vi "Testing Mode.vi"(8 "Filepath":path=path "D:/My Project/2019-2020/Magnetic Mareli UM/MM_UM/Project Setup/data/program seq/Program_280A.bin", 9 "FeedBack Channel":string[](array[string])=["fgdgfvcbc", "vnfhgjkn", "21354682"]) -> ()   [LabVIEW 2015]
uses:
  Control Button/Exit.ctl
  Control Button/Start.ctl
  Test  enqueue/AutoTest seq.ctl
  Test  enqueue/Auot Test selection.ctl
  Galobal variable_TI.vi
  Project Setup/Globle Variable/GR_Servo.vi
  <vilib>/Utility/file.llb/Write Delimited Spreadsheet (string).vi
panel:
  out "Ready":bool
  in  "Seq1":enum16{"Seq_1", "Seq_2", "Seq_3", "Seq_4"}(ring)
  out "Dist. data":dbl[](array[numeric]) format="%0.03f"
  out "Proxi Sensor":bool
  in  "value":bool
  out "reset":bool
  out "D-enqueue":T1
  out "Servo Fault":bool
  in  "Report":bool
  out "Start":bool
  in  "Cycle":i32
  in  "Home Call":bool
  out "DI":bool[](array[boolean])
  out "Current Date & Time":timestamp
  in  "Cycle Start Bit":bool
  in  "vi reference":refnum<vi>
  in  "Reset Ct.":bool
  out "error out":errorcluster
  in  "Tbl Refnum":refnum<vi>
  in  "Tab Control":enum32{"Test", "Report"}(tab)
  out "RR":bool
  out "RL":bool
  out "FR":bool
  out "FL":bool
  out "Error Message 2":string
  out "User Name":string
  out "Error Message":string
  out "Running Model":string
  out "Date time":string
  out "MIC Barcode":string
  out "2D Picture":picture
  out "Screw Data(N)":T2
  in  "Tab Control 2":enum32{"TESTING", "HOME"}(tab)
  in  "Table Control":string[][](table)
  in  "home":string[][](table)
  out "Error":bool
  out "Read LVDT Value":dbl[](array[numeric]) format="%0.03f"
  out "Result Lvdt 2":T3 {"Screw4(mm)" format="%0.02f"; "Screw3(mm)" format="%0.02f"; "Screw 2(mm)" format="%0.02f"; "Screw1(mm)" format="%0.02f"}
  out "Result Lvdt":T4
  out "Test Name":string
  in  "Exit":T5
  in  "Start 2":T6
  out "Cycle Time(Sec)":i32
  out "MIC Code":string
  in  "OK Counter":string
  in  "NG Counter":string
  in  "RPT Bypass":bool=TRUE
  out "Pokayoka":T7
  out "Boolean 2":bool
  in  "Report":i32(listbox)
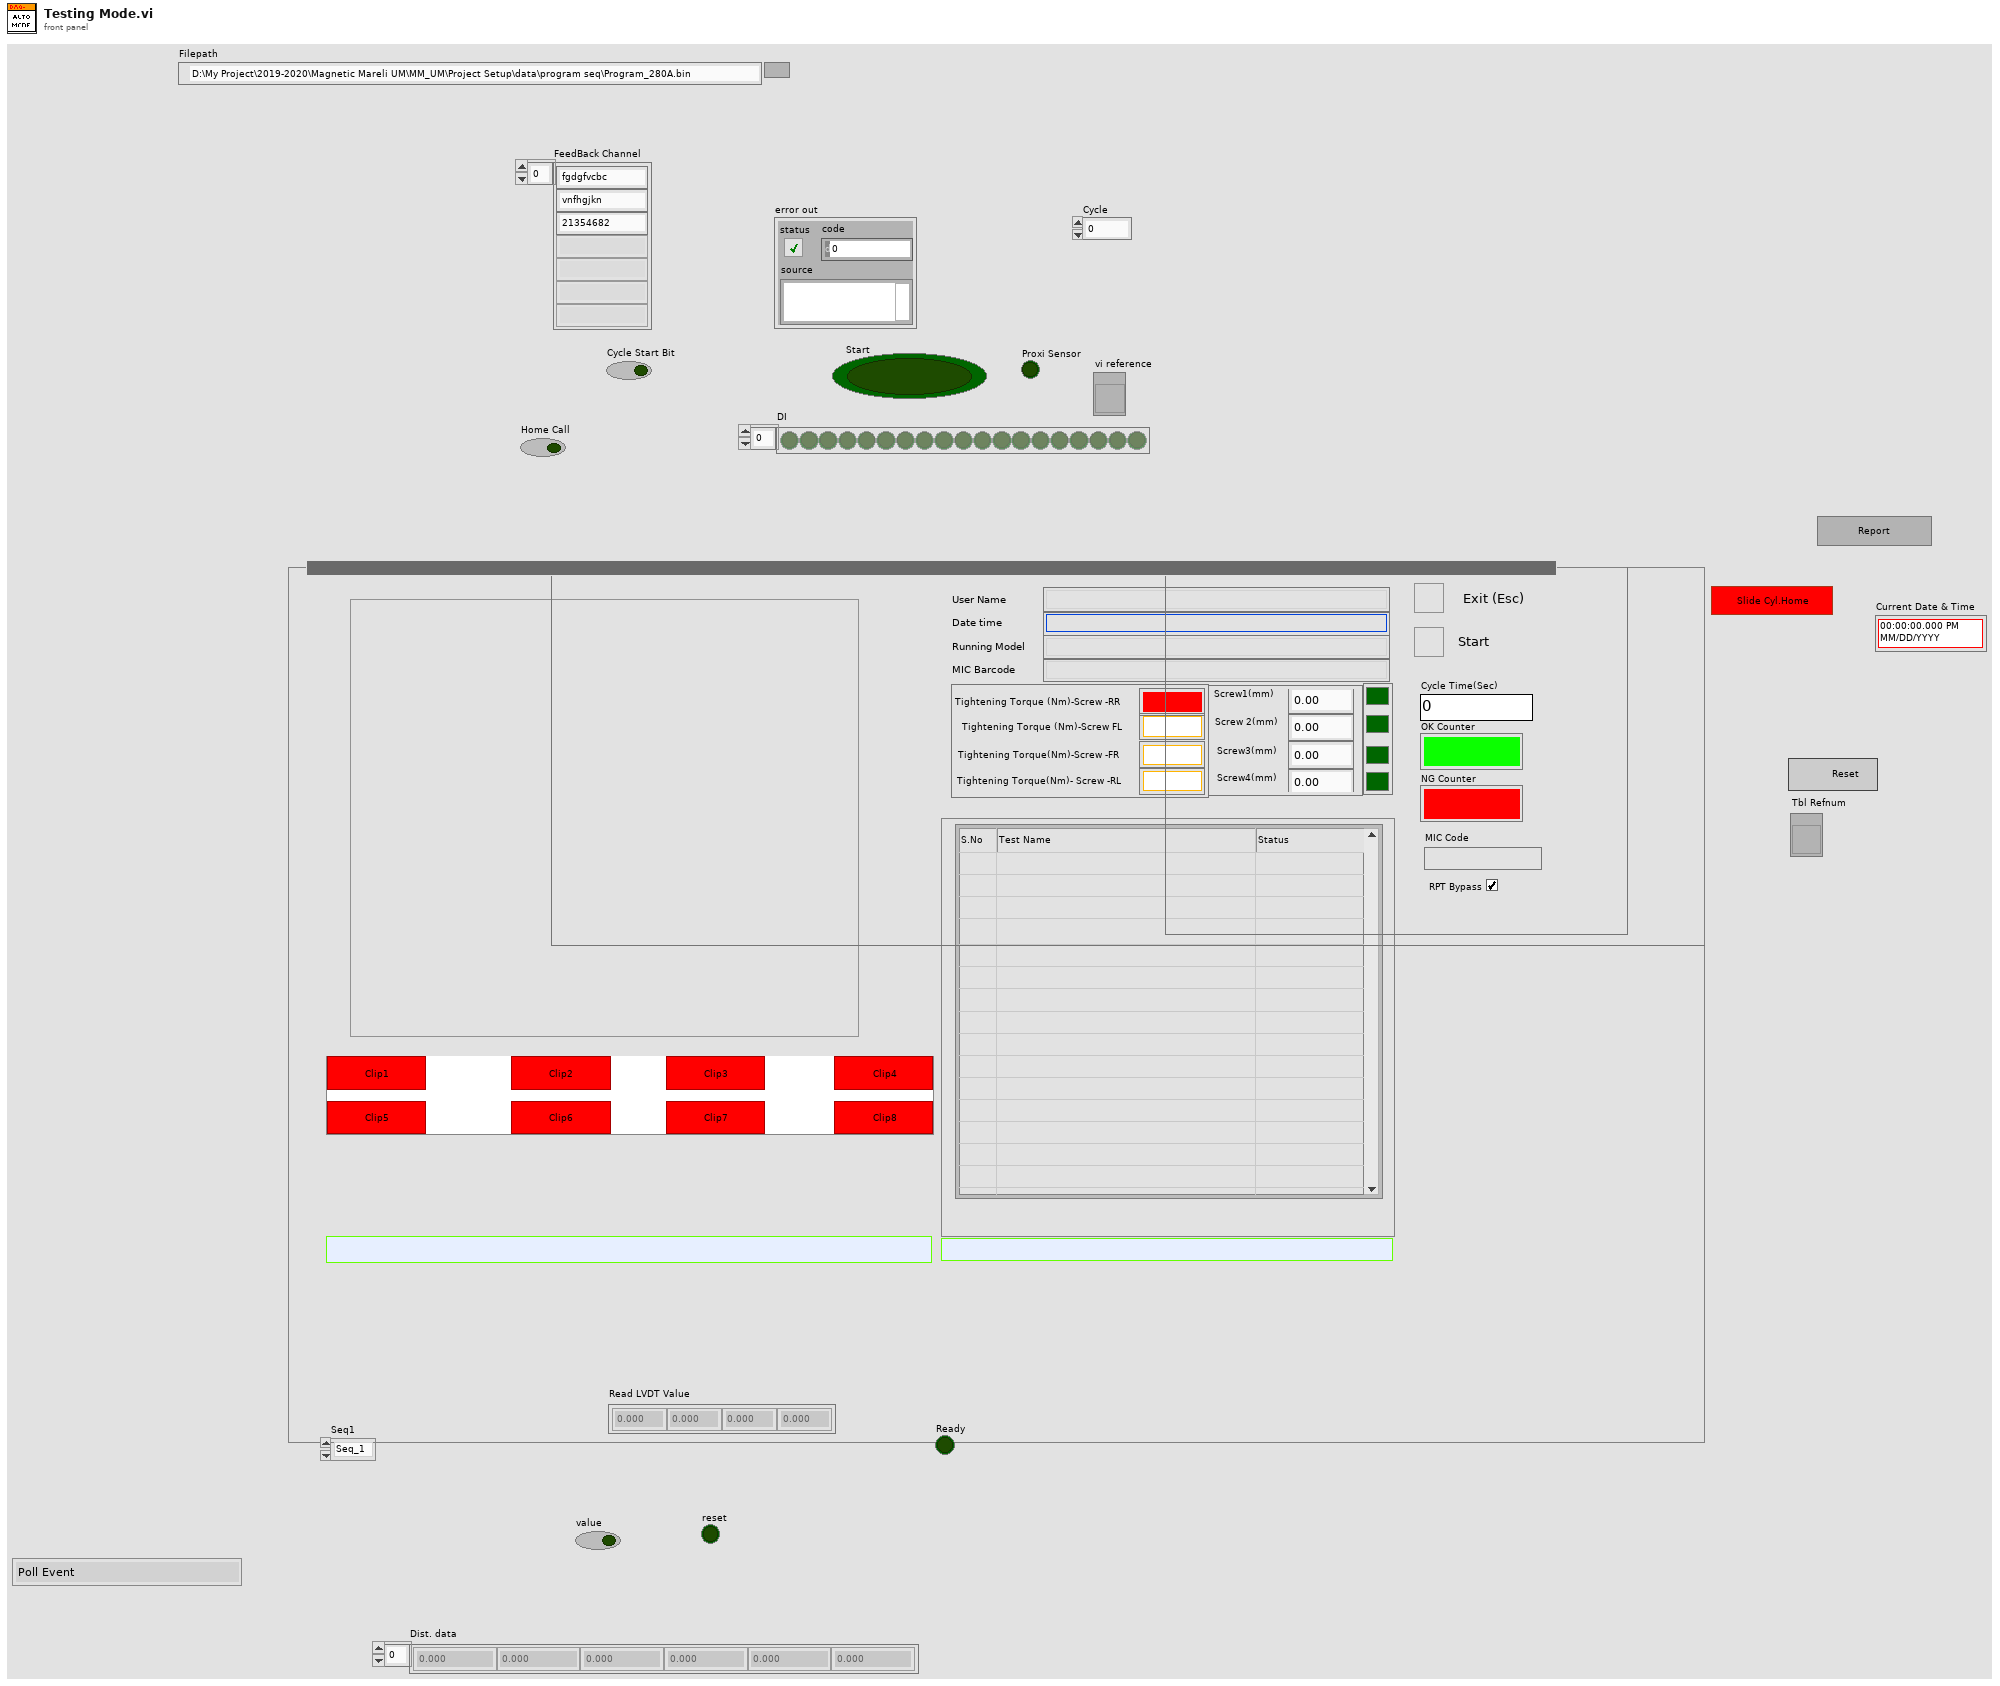
[diagram p1: front panel]
types:
  T1 = typedef "AutoTest seq.ctl" = enum16{"Poll Event", "Part Clamp", "Program Seq", "Cylender Home", "Result Save", "Error", "Exit"}
  T2 = cluster{"Tightening Torque (Nm)-Screw -RR":string, "Tightening Torque (Nm)-Screw FL ":string, "Tightening Torque(Nm)-Screw -FR":string, "Tightening Torque(Nm)- Screw -RL":string}
  T3 = cluster{"Screw1(mm)":dbl, "Screw 2(mm)":dbl, "Screw3(mm)":dbl, "Screw4(mm)":dbl}
  T4 = cluster{"Screw Height-1":bool, "Screw Height-2":bool, "Screw Height-3":bool, "Screw Height-4":bool}
  T5 = typedef "Exit.ctl" = bool
  T6 = typedef "Start.ctl" = bool
  T7 = cluster{"Clip1":bool, "Clip2 3":bool, "Clip3 3":bool, "Clip4":bool, "Clip5":bool, "Clip6":bool, "Clip7":bool, "Clip8":bool}
  T8 = cluster{"Screw -FL":string, "Screw -FR":string, "Screw -RL":string, "Screw -RR":string}
  T9 = cluster{"MIC ":refnum<visa-resource-name>, "baud rate MIC ":u32, "LCD ":refnum<visa-resource-name>, "baud rate_LCD":u32}
  T10 = typedef "Auot Test selection.ctl" = enum16{"Init", "Enqueue ", "Enqueue N", "Enqueue in stack", "Enqueue in stack N", "Dequeue", "Dequeue N", "Flush", "Release Queue"}
  T11 = cluster{"LVDT1Max(mm) AI0":dbl, "LVDT1Min (mm)AI0":dbl, "LVDT2Max(mm) AI1":dbl, "LVDT2Min(mm) AI1":dbl, "LVDT3Max(mm) AI2":dbl, "LVDT3Min(mm) AI2":dbl, "LVDT4Max(mm) AI3":dbl, "LVDT4Min(mm) AI3":dbl, "Model":string, "MIC Code":string}
  T12 = cluster{"Item Name":string, "Item Status":bool, "Steps":cluster{"Channel Type":string, "Channels":string, "Wait/Poll (ms)":u32, "Parameter":u8, "STM-Speed":i32, "STM-Degree":u32, "Direction":u8}[]}[]
  T13 = cluster{"Nuth Height1":bool, "Nuth Height2":bool, "Nuth Height3":bool, "Nuth Height4":bool}
  T14 = enum16{"Part Clamp", "Part Unclamp", "Part Clamp Input Check", "Part Unclamp Input Check"}
  T15 = cluster{"No. Fail Coun t":string, "Rework Status Count 0\\1":string, "NA Count Max =3 ":string, "Testesd Count  0/1":string, "Error code":string}
  T16 = cluster{"Emergency_1":bool, "Reset_2":bool, "Air Pressure_4":bool, "Safety Sensor_5":bool, "Safety Sensor_6":bool, "Barcode Rev rs_24":bool, "Clamp fwd rs_21":bool, "Servo Fault":bool, "Home _3":bool}
  T17 = cluster{"Read LVDT Value[0]":dbl, "Read LVDT Value[1]":dbl, "Read LVDT Value[2]":dbl, "Read LVDT Value[3]":dbl}
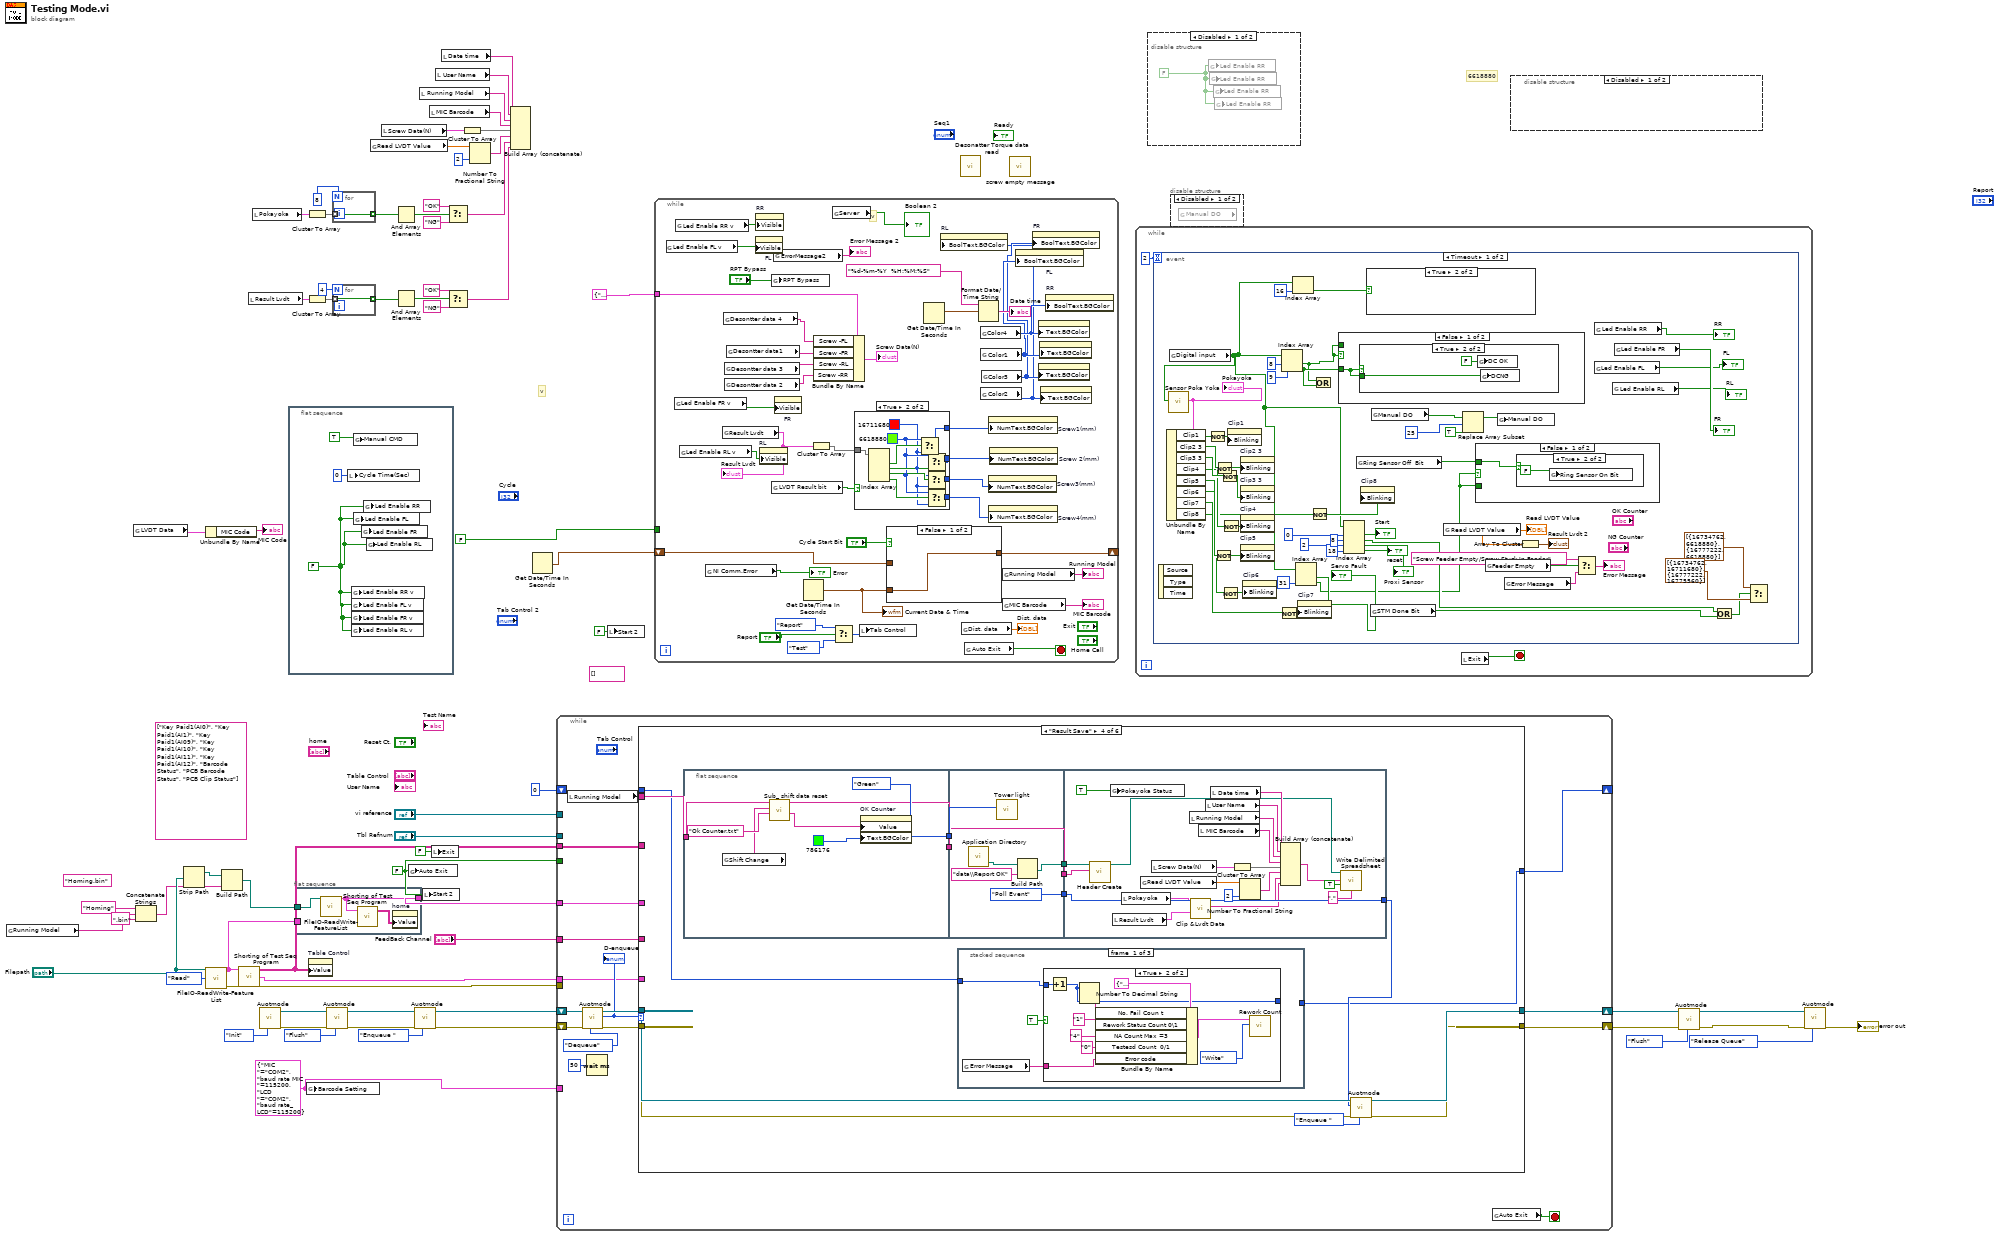
[diagram p0: block diagram]
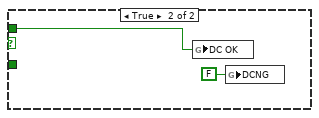
[diagram p7: hidden frame]
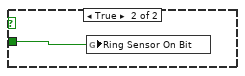
[diagram p9: hidden frame]
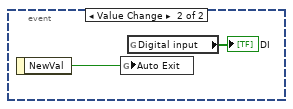
[diagram p10: hidden frame]
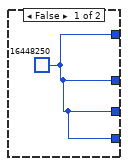
[diagram p11: hidden frame]
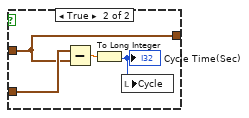
[diagram p12: hidden frame]
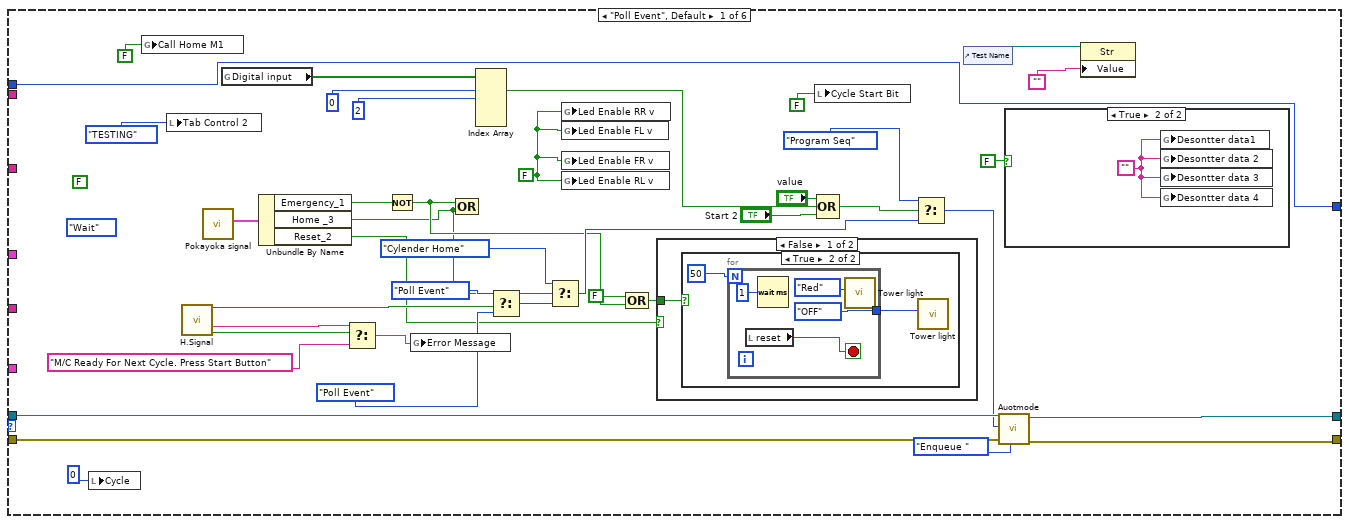
[diagram p13: hidden frame]
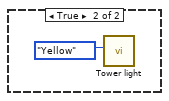
[diagram p16: hidden frame]
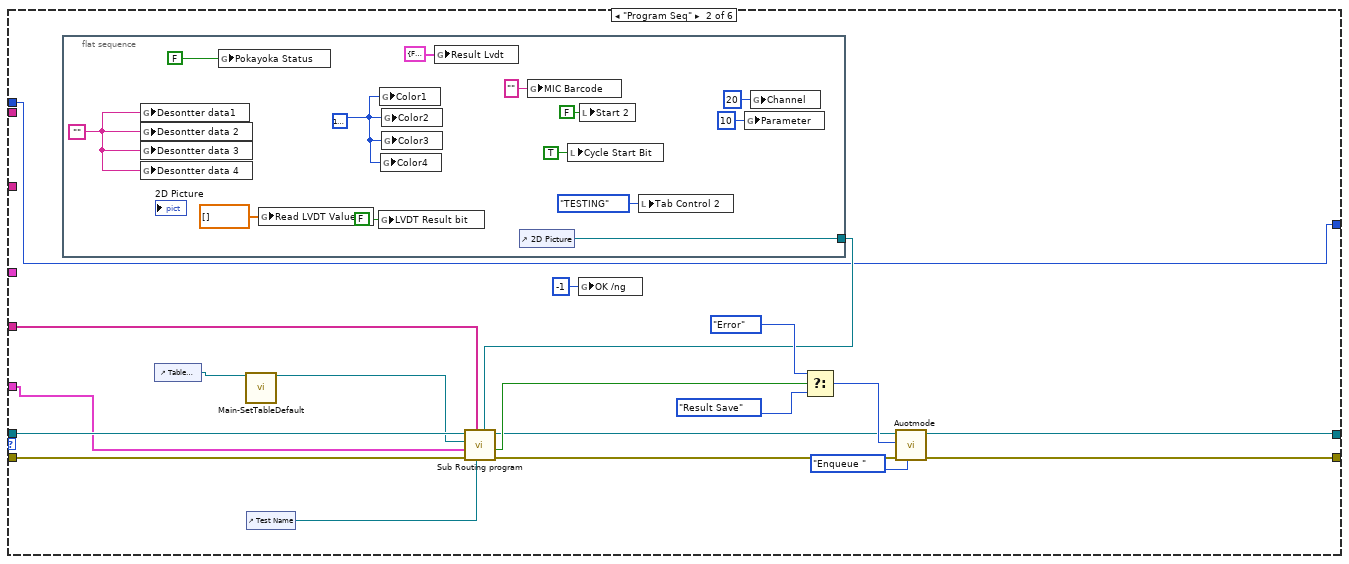
[diagram p17: hidden frame]
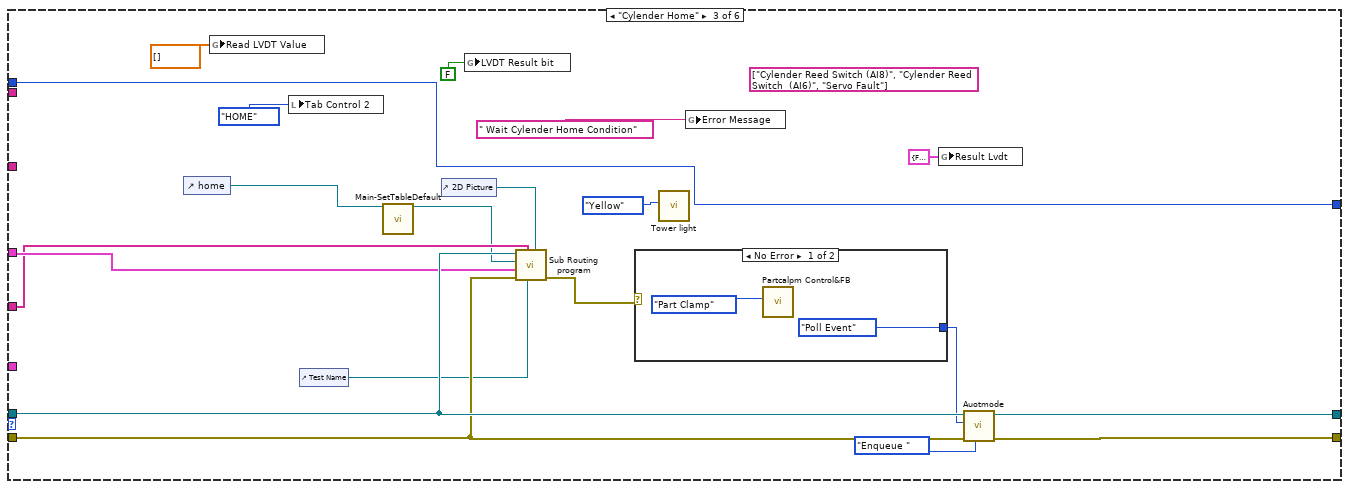
[diagram p18: hidden frame]
diagram:
  w34 = T9 {"MIC "="COM2", "baud rate MIC "=115200, "LCD "="COM2", "baud rate_LCD"=115200} ("Barcode Setting")
  (unwired) "Homing.bin" ("name or relative path")
  (unwired) string[] ["Key Paid1(AI0)", "Key Paid1(AI1)", "Key Paid1(AI09)", "Key Paid1(AI10)", "Key Paid1(AI11)", "Key Paid1(AI12)", "Barcode Status", "PCB Barcode Status", "PCB Clip Status"] ("Error Name")
  (unwired) string[] []
  w41 = FALSE ("Auto Exit")
  # "v"
  # "6618880"
  n1 = global read "Galobal variable_TI.vi" "Running Model"() -> (w32:string)
  n2 = global read "Galobal variable_TI.vi" "LVDT Data"() -> (w28:T11)
  n3 = Concatenate Strings("Homing" ("string"), w32, ".bin" ("string")) -> (w30:string)
  n4 = Strip Path(path="Filepath") -> (stripped path=w38:path)  [unwired: 1 out]
  n5 = Unbundle By Name(w28) -> ("MIC Code"=→"MIC Code":string)
  n6 = call "FileIO-ReadWrite-FeatureList.vi"("Filepath"="Filepath", "Read/Write"=enum16{"Read", "Write"}."Read") -> ("Feature List (Out)"=w36:T12, "Error Out"=w49:errorcluster)  [unwired: 12 in]
  n7 = Build Path(base path=w38, name or relative path=w30) -> (appended path=w37:path)
  n8 = call "Shorting of Test Seq Program.vi"("Feature List (Out)"=w36) -> ("Feature Step Enable"=w43:T12, "Feature Name"=w42:string[][])  [unwired: 3 in]
  n9 = local read "Result Lvdt"() -> (w9:T4)
  n10 = local read "Pokayoka"() -> (w17:T7)
  n11 = call "Auotmode.vi"("Enum Selection"=Auot_Test_selection."Init") -> ("error out"=w61:errorcluster, "queue Out"=w59:refnum<queue>)  [unwired: 7 in, 1 out]
  n12 = flat-sequence {
    frame #0 {
      w68 = FALSE ("RPT Bypass")
      n13 = local write "Cycle Time(Sec)"(0 ("Cycle Time(Sec)")) -> ()
      n14 = global write "Galobal variable_TI.vi" "Led Enable RR v"(w68) -> ()
      n15 = global write "Galobal variable_TI.vi" "Led Enable FL v"(w68) -> ()
      n16 = global write "Galobal variable_TI.vi" "Led Enable FR v"(w68) -> ()
      n17 = global write "Galobal variable_TI.vi" "Led Enable RL v"(w68) -> ()
      n18 = global write "Galobal variable_TI.vi" "Manual CMD"(TRUE ("Manual CMD")) -> ()
      n19 = global write "Galobal variable_TI.vi" "Led Enable FL"(w68) -> ()
      n20 = global write "Galobal variable_TI.vi" "Led Enable FR"(w68) -> ()
      n21 = global write "Galobal variable_TI.vi" "Led Enable RR"(w68) -> ()
      n22 = global write "Galobal variable_TI.vi" "Led Enable RL"(w68) -> ()
    }
  }
  n23 = flat-sequence {
    tunnel: w37 -> [w73]
    tunnel: w36 -> [_]
    tunnel: [w72] -> w35
    frame #0 {
      n24 = call "FileIO-ReadWrite-FeatureList.vi"("Filepath"=w73) -> ("Feature List (Out)"=w72:T12)  [unwired: 13 in, 1 out]
      n25 = call "Shorting of Test Seq Program.vi"("Feature List (Out)"=w72) -> ("Feature Name"=w71:string[][])  [unwired: 3 in, 1 out]
      n26 = property on="home" class="Tbl (strict)"("Value"=w71) -> ()  [unwired: 2 in, 2 out]
    }
  }
  n27 = Cluster To Array(cluster=w17) -> (array=w16:bool[])
  n28 = Cluster To Array(cluster=w9) -> (array=w8:bool[])
  n29 = global write "Galobal variable_TI.vi" "Barcode Setting"(w34) -> ()
  n30 = property on="Table Control" class="Tbl (strict)"("Value"=w42) -> ()  [unwired: 2 in, 2 out]
  n31 = call "Auotmode.vi"("Enum Selection"=Auot_Test_selection."Flush", "Error In"=w61, "queue in"=w59) -> ("error out"=w60:errorcluster, "queue Out"=w58:refnum<queue>)  [unwired: 5 in, 1 out]
  n32 = for {
    N: 8 -> [_]
    tunnel: w16 -> [w74] mode=indexing
    tunnel: [w74] -> w14 mode=indexing
  }
  n33 = for {
    N: 4 -> [_]
    tunnel: w8 -> [w75] mode=indexing
    tunnel: [w75] -> w4 mode=indexing
  }
  n34 = global read "Galobal variable_TI.vi" "Read LVDT Value"() -> (w20:dbl[])
  n35 = local read "Screw Data(N)"() -> (w22:T2)
  n36 = And Array Elements(Boolean array=w14) -> (logical AND=w13:bool)
  n37 = And Array Elements(Boolean array=w4) -> (logical AND=w5:bool)
  n38 = global write "Galobal variable_TI.vi" "Auto Exit"(w41) -> ()
  n39 = call "Auotmode.vi"("Enum Selection"=Auot_Test_selection."Enqueue ", "Error In"=w60, "queue in"=w58) -> ("error out"=w65:errorcluster, "queue Out"=w46:refnum<queue>)  [unwired: 5 in, 1 out]
  n40 = local read "Running Model"() -> (w24:string)
  n41 = local write "Start 2"(w41) -> ()
  n42 = local read "MIC Barcode"() -> (w23:string)
  n43 = local write "Exit"(T5 FALSE ("Exit")) -> ()
  n44 = local read "User Name"() -> (w25:string)
  n45 = local read "Date time"() -> (w26:string)
  n46 = Select(t="OK" ("Screw -FL"), s=w13, f="NG" ("Screw -FL")) -> (s? t:f=w10:string)
  n47 = Select(t="OK" ("Screw -FL"), s=w5, f="NG" ("Screw -FL")) -> (s? t:f=w3:string)
  n48 = Cluster To Array(cluster=w22) -> (array=w21:string[])
  n49 = Number To Fractional String(number=w20, precision (6)=i16 2) -> (F-format string=w18:string[])  [unwired: 2 in]
  n50 = Build Array (concatenate)(w26, w25, w24, w23, w21, w18, w10, w3) -> ()  [unwired: 1 out]
  n51 = Get Date/Time In Seconds() -> (seconds since 1Jan1904=w51:timestamp)
  n52 = while {
    tunnel: "vi reference" -> [_]
    tunnel: "Tbl Refnum" -> [_]
    tunnel: w43 -> [w85]
    tunnel: w49 -> [_]
    tunnel: "FeedBack Channel" -> [w86]
    shift-right: [w89] -> w52
    shift-left: w46 -> [w82]
    shift-right: [w81] -> w45
    shift-left: w65 -> [w91]
    tunnel: w41 -> [_]
    tunnel: w42 -> [w80]
    tunnel: w35 -> [w78]
    tunnel: w34 -> [_]
    shift-right: [w76] -> _
    shift-left: 0 -> [w77]
    stop <- w84 stop-if-true
    n53 = local read "Running Model"() -> (w79:string)
    n54 = call "Auotmode.vi"("Enum Selection"=Auot_Test_selection."Dequeue", "Error In"=w91, "queue in"=w82) -> ("error out"=w88:errorcluster, "D-enqueue"=w87:T1, "queue Out"=w90:refnum<queue>)  [unwired: 5 in]
    "D-enqueue" <- w87
    n55 = Wait (ms)(milliseconds to wait=u32 50) -> ()  [unwired: 1 out]
    n56 = case shown="\"Result Save\"" w87 {
      tunnel: w90 -> [w132 w150 w190 w208 w273 w343]
      tunnel: [w130 w156 w192 w206 w272 w344] -> w89
      tunnel: w88 -> [w131 w152 w189 w207 w271 w345]
      tunnel: [w129 w155 w191 w205 w270 w345] -> w81
      tunnel: w85 -> [_ w145 _ _ _ _]
      tunnel: w86 -> [_ w153 w187 _ _ _]
      tunnel: w80 -> [_ _ _ _ _ _]
      tunnel: w79 -> [_ _ _ w204 w264 _]
      tunnel: w78 -> [_ _ w188 _ _ _]
      tunnel: w77 -> [w93 w142 w174 w197 w261 w321]
      tunnel: [w93 w142 w174 w196 w260 w321] -> w76
      frame "Poll Event", Default {
        w94 = FALSE
        (unwired) enum16{"Wait", "Ionizer On", "Ionizer off"}."Wait" ("Enum")
        (unwired) FALSE ("Ionizer cnf")
        n57 = local write "Cycle"(0 ("Cycle")) -> ()
        n58 = global write "Galobal variable_TI.vi" "Call Home M1"(FALSE ("Call Home M1")) -> ()
        n59 = local write "Tab Control 2"(enum32{"TESTING", "HOME"}."TESTING" ("Tab Control 2")) -> ()
        n60 = call "H.Signal.vi"() -> ("Slide servo home RS"=w117:bool, "Error Message"=w118:string, "Bool_H Sig"=w101:bool)  [unwired: 10 in, 3 out]
        n61 = call "Pokayoka signal.vi"() -> ("output cluster"=w111:T16)  [unwired: 10 in, 1 out]
        n62 = global read "Galobal variable_TI.vi" "Digital input"() -> (w127:bool[])
        n63 = Unbundle By Name(w111) -> ("Emergency_1"=w110:bool, "Home _3"=w97:bool, "Reset_2"=w103:bool)
        n64 = Select(t=w118, s=w101, f="M/C Ready For Next Cycle. Press Start Button") -> (s? t:f=w104:string)
        n65 = Not(x=w110) -> (.not. x?=w105:bool)
        n66 = global write "GR_Servo.vi" "Error Message"(w104) -> ()
        n67 = Compound Arithmetic op=OR(w105, w97) -> ()  [unwired: 1 out]
        n68 = Index Array(array=w127, index #1=0 ("index"), index #2=2 ("index")) -> (element #1=w112:bool)  [unwired: 3 in, 4 out]
        n69 = Select(t=AutoTest_seq."Poll Event" ("Enqueue"), s=w117, f=AutoTest_seq."Poll Event") -> (s? t:f=w122:T1)
        n70 = Select(t=AutoTest_seq."Cylender Home" ("Enqueue"), s=w97, f=w122) -> (s? t:f=w109:T1)
        n71 = global write "Galobal variable_TI.vi" "Led Enable RR v"(w94) -> ()
        n72 = global write "Galobal variable_TI.vi" "Led Enable FL v"(w94) -> ()
        n73 = global write "Galobal variable_TI.vi" "Led Enable FR v"(w94) -> ()
        n74 = global write "Galobal variable_TI.vi" "Led Enable RL v"(w94) -> ()
        n75 = Compound Arithmetic op=OR(FALSE ("value"), w105) -> (w102:bool)
        n76 = case shown="False" w103 {
          tunnel: w102 -> [w134 _]
          frame False {
            n77 = case shown="True" w134 {
              frame False {
              }
              frame True {
                n78 = for {
                  N: 50 -> [_]
                  tunnel: [enum16{"Green", "Red", "Yellow", "OFF"}."OFF" ("Enum")] -> w135
                  stop <- w137 stop-if-true
                  n79 = local read "reset"() -> (w137:bool)
                  n80 = Wait (ms)(milliseconds to wait=u32 1) -> ()  [unwired: 1 out]
                  n81 = call "Tower light.vi"("Enum"=enum16{"Green", "Red", "Yellow"}."Red") -> ()  [unwired: 11 in]
                }
                n82 = call "Tower light.vi"("Enum"=w135) -> ()  [unwired: 11 in]
              }
            }
          }
          frame True {
            n83 = call "Tower light.vi"("Enum"=enum16{"Green", "Red", "Yellow"}."Yellow") -> ()  [unwired: 11 in]
          }
        }
        n84 = local write "Cycle Start Bit"(FALSE ("Cycle Start Bit")) -> ()
        n85 = Compound Arithmetic op=OR("value", w112, "Start 2") -> (w96:T6)
        n86 = Select(t=AutoTest_seq."Program Seq" ("Enqueue"), s=w96, f=w109) -> (s? t:f=w108:T1)
        n87 = control-ref of="Test Name"() -> (w107:refnum<vi>)
        n88 = call "Auotmode.vi"("Enum Selection"=Auot_Test_selection."Enqueue ", "Error In"=w131, "Enqueue"=w108, "queue in"=w132) -> ("error out"=w129:errorcluster, "queue Out"=w130:refnum<queue>)  [unwired: 4 in, 1 out]
        n89 = case shown="True" FALSE {
          frame False {
          }
          frame True {
            w133 = ""
            n90 = global write "Galobal variable_TI.vi" "Desontter data1"(w133) -> ()
            n91 = global write "Galobal variable_TI.vi" "Desontter data 2"(w133) -> ()
            n92 = global write "Galobal variable_TI.vi" "Desontter data 3"(w133) -> ()
            n93 = global write "Galobal variable_TI.vi" "Desontter data 4"(w133) -> ()
          }
        }
        n94 = property class="Str"(reference=w107, "Value"="") -> ()  [unwired: 1 in, 2 out]
      }
      frame "Program Seq" {
        n95 = flat-sequence {
          tunnel: [w161] -> w143
          frame #0 {
            w168 = u32 16777226 ("Color Box")
            w169 = ""
            n96 = global write "Galobal variable_TI.vi" "Desontter data1"(w169) -> ()
            n97 = global write "Galobal variable_TI.vi" "Desontter data 2"(w169) -> ()
            n98 = global write "Galobal variable_TI.vi" "Desontter data 3"(w169) -> ()
            n99 = global write "Galobal variable_TI.vi" "Desontter data 4"(w169) -> ()
            n100 = global write "Galobal variable_TI.vi" "Pokayoka Status"(FALSE ("Rpt Write")) -> ()
            n101 = global write "Galobal variable_TI.vi" "Read LVDT Value"(dbl[] [] ("Read LVDT Value")) -> ()
            n102 = global write "Galobal variable_TI.vi" "LVDT Result bit"(FALSE ("LVDT Result bit")) -> ()
            n103 = global write "Galobal variable_TI.vi" "Color1"(w168) -> ()
            n104 = global write "Galobal variable_TI.vi" "Color4"(w168) -> ()
            n105 = global write "Galobal variable_TI.vi" "Color2"(w168) -> ()
            n106 = global write "Galobal variable_TI.vi" "Color3"(w168) -> ()
            n107 = global write "Galobal variable_TI.vi" "Result Lvdt"(T13 {"Nuth Height1"=FALSE, "Nuth Height2"=FALSE, "Nuth Height3"=FALSE, "Nuth Height4"=FALSE} ("Result Lvdt")) -> ()
            n108 = control-ref of="2D Picture"() -> (w161:refnum<vi>)
            n109 = global write "Galobal variable_TI.vi" "MIC Barcode"("" ("MIC Barcode")) -> ()
            n110 = local write "Cycle Start Bit"(TRUE ("Cycle Start Bit")) -> ()
            n111 = local write "Start 2"(T6 FALSE ("Start")) -> ()
            n112 = local write "Tab Control 2"(enum32{"TESTING", "HOME"}."TESTING" ("Tab Control 2")) -> ()
            n113 = global write "Galobal variable_TI.vi" "Parameter"(u8 10 ("Parameter")) -> ()
            n114 = global write "Galobal variable_TI.vi" "Channel"(20 ("Channel")) -> ()
          }
        }
        n115 = control-ref of="Table Control"() -> (w147:refnum<vi>)
        n116 = call "Main-SetTableDefault.vi"("Table (In)"=w147) -> ("Table (Out)"=w146:refnum<vi>)  [unwired: 13 in, 1 out]
        n117 = control-ref of="Test Name"() -> (w148:refnum<vi>)
        n118 = call "Sub Routing program.vi"("Image"=w143, "Test Name"=w148, "FeedBack Channel"=w153, "error in (no error)"=w152, "Feature Step Enable"=w145, "Table"=w146, "queue Out in"=w150) -> ("error out"=w151:errorcluster, "Error"=w154:bool, "Queue out"=w149:refnum<queue>)  [unwired: 1 in, 1 out]
        n119 = global write "Galobal variable_TI.vi" "OK /ng"(-1 ("OK /ng")) -> ()
        n120 = Select(t=AutoTest_seq."Error" ("Enqueue"), s=w154, f=AutoTest_seq."Result Save" ("Enqueue")) -> (s? t:f=w157:T1)
        n121 = call "Auotmode.vi"("Enum Selection"=Auot_Test_selection."Enqueue ", "Error In"=w151, "Enqueue"=w157, "queue in"=w149) -> ("error out"=w155:errorcluster, "queue Out"=w156:refnum<queue>)  [unwired: 4 in, 1 out]
      }
      frame "Cylender Home" {
        (unwired) string[] ["Cylender Reed Switch (AI8)", "Cylender Reed Switch  (AI6)", "Servo Fault"]
        n122 = control-ref of="home"() -> (w178:refnum<vi>)
        n123 = global write "Galobal variable_TI.vi" "Read LVDT Value"(dbl[] [] ("Read LVDT Value")) -> ()
        n124 = local write "Tab Control 2"(enum32{"TESTING", "HOME"}."HOME" ("Tab Control 2")) -> ()
        n125 = control-ref of="Test Name"() -> (w186:refnum<vi>)
        n126 = call "Main-SetTableDefault.vi"("Table (In)"=w178) -> ("Table (Out)"=w184:refnum<vi>)  [unwired: 13 in, 1 out]
        n127 = control-ref of="2D Picture"() -> (w185:refnum<vi>)
        n128 = global write "Galobal variable_TI.vi" "LVDT Result bit"(FALSE ("LVDT Result bit")) -> ()
        n129 = call "Sub Routing program.vi"("Image"=w185, "Test Name"=w186, "FeedBack Channel"=w187, "error in (no error)"=w189, "Feature Step Enable"=w188, "Table"=w184, "queue Out in"=w190) -> ("error out"=w181:errorcluster)  [unwired: 1 in, 3 out]
        n130 = case shown="No Error" w181 {
          tunnel: [AutoTest_seq."Poll Event" ("Enqueue") _] -> w180
          frame No Error {
            n131 = call "Partcalpm Control&FB.vi"("Enum"=T14."Part Clamp") -> ()  [unwired: 9 in, 2 out]
          }
          frame Error {
          }
        }
        n132 = call "Tower light.vi"("Enum"=enum16{"Green", "Red", "Yellow"}."Yellow") -> ()  [unwired: 11 in]
        n133 = global write "GR_Servo.vi" "Error Message"(" Wait Cylender Home Condition") -> ()
        n134 = global write "Galobal variable_TI.vi" "Result Lvdt"(T13 {"Nuth Height1"=FALSE, "Nuth Height2"=FALSE, "Nuth Height3"=FALSE, "Nuth Height4"=FALSE} ("Result Lvdt")) -> ()
        n135 = call "Auotmode.vi"("Enum Selection"=Auot_Test_selection."Enqueue ", "Error In"=w189, "Enqueue"=w180, "queue in"=w190) -> ("error out"=w191:errorcluster, "queue Out"=w192:refnum<queue>)  [unwired: 4 in, 1 out]
      }
      frame "Result Save" {
        n136 = flat-sequence {
          tunnel: w204 -> [w228]
          tunnel: [enum16{"Green", "Red", "Yellow"}."Green" ("Enum")] -> w203
          tunnel: [w228] -> w199
          tunnel: w203 -> [w238]
          tunnel: [AutoTest_seq."Poll Event" ("Enqueue")] -> w201
          tunnel: [w236] -> w200
          tunnel: w199 -> [w236]
          tunnel: [w233] -> w198
          tunnel: [w259] -> w202
          tunnel: w201 -> [w259]
          tunnel: w200 -> [w258]
          tunnel: w198 -> [w257]
          frame #0 {
            n137 = global read "Galobal variable_TI.vi" "Shift Change"() -> (w227:string)
            n138 = call "Sub_ shift data reset.vi"("Serial no"="Ok Counter.txt" ("File Name"), "Shift"=w227, "Model"=w228) -> ("Serial no"=w231:string)  [unwired: 6 in, 1 out]
            n139 = property on="OK Counter" class="Str"("Value"=w231, "Text.BGColor"=u32 786176 ("Color Box")) -> ()  [unwired: 2 in, 2 out]
          }
          frame #1 {
            n140 = call <vilib>:"Application Directory.vi"() -> ("Application Directory"=w235:path)
            n141 = call "Tower light.vi"("Enum"=w238) -> ()  [unwired: 11 in]
            n142 = Build Path(base path=w235, name or relative path="data\\Report OK") -> (appended path=w233:path)
          }
          frame #2 {
            n143 = call "Header Create.vi"("File Name"=w258, "path File"=w257) -> ("dup path"=w244:path)  [unwired: 8 in, 1 out]
            n144 = global write "Galobal variable_TI.vi" "Pokayoka Status"(TRUE ("Rpt Write")) -> ()
            n145 = local read "Result Lvdt"() -> (w247:T4)
            n146 = local read "Pokayoka"() -> (w239:T7)
            n147 = global read "Galobal variable_TI.vi" "Read LVDT Value"() -> (w250:dbl[])
            n148 = local read "Screw Data(N)"() -> (w252:T2)
            n149 = local read "Running Model"() -> (w254:string)
            n150 = call "Clip &Lvdt Data.vi"("Pokayoka"=w239, "Result Lvdt in"=w247) -> ("Clip Status"=w246:string, "Screw Height Status"=w245:string)  [unwired: 7 in]
            n151 = local read "MIC Barcode"() -> (w253:string)
            n152 = local read "User Name"() -> (w255:string)
            n153 = local read "Date time"() -> (w256:string)
            n154 = Cluster To Array(cluster=w252) -> (array=w251:string[])
            n155 = Number To Fractional String(number=w250, precision (6)=i16 2) -> (F-format string=w248:string[])  [unwired: 2 in]
            n156 = Build Array (concatenate)(w256, w255, w254, w253, w251, w248, w246, w245) -> (w243:string[])
            n157 = call-poly <vilib>:"Write Delimited Spreadsheet.vi"("file path (dialog if empty)"=w244, "1D data"=w243, "append to file? (F)"=TRUE, "delimiter (\\t)"="," ("delimiter (\\t)")) -> ()  [unwired: 10 in, 2 out]
          }
        }
        n158 = stacked-sequence {
          tunnel: w197 -> [w212 _ _]
          tunnel: [_ _ 0] -> w196
          frame #0 {
            n159 = global read "GR_Servo.vi" "Error Message"() -> (w211:string)
            n160 = case shown="True" TRUE {
              tunnel: w212 -> [w213 w222]
              tunnel: w211 -> [_ w217]
              tunnel: [w213 w214] -> _
              frame False {
              }
              frame True {
                n161 = Increment(x=w222) -> (x+1=w214:i32)
                n162 = Number To Decimal String(number=w214) -> (decimal integer string=w221:string)  [unwired: 1 in]
                n163 = Bundle By Name(cluster=T15 {"No. Fail Coun t"="", "Rework Status Count 0\\1"="", "NA Count Max =3 "="", "Testesd Count  0/1"="", "Error code"=""} ("Count For Rework"), "No. Fail Coun t"=w221, "Rework Status Count 0\\1"="1" ("Rework Status Count 0\\1"), "NA Count Max =3"="4", "Testesd Count  0/1"="0", "Error code"=w217) -> (w216:T15)
                n164 = call "Rework Count.vi"("Read /Write"=enum16{"Write", "Read"}."Write", "Count For Rework"=w216) -> ()  [unwired: 8 in, 2 out]
              }
            }
          }
          frame #1 {
            n165 = Wait (ms)(milliseconds to wait=u32 200) -> ()  [unwired: 1 out]
          }
          frame #2 {
            n166 = global write "Galobal variable_TI.vi" "Rpt Write"(TRUE ("Rpt Write")) -> ()
          }
        }
        n167 = call "Auotmode.vi"("Enum Selection"=Auot_Test_selection."Enqueue ", "Error In"=w207, "Enqueue"=w202, "queue in"=w208) -> ("error out"=w205:errorcluster, "queue Out"=w206:refnum<queue>)  [unwired: 4 in, 1 out]
      }
      frame "Error" {
        n168 = call "Pokayoka signal.vi"() -> ("output cluster"=w268:T16)  [unwired: 10 in, 1 out]
        n169 = Unbundle By Name(w268) -> ("Home _3"=w262:bool)
        n170 = call "Tower light.vi"("Enum"=enum16{"Green", "Red", "Yellow"}."Red") -> ()  [unwired: 11 in]
        n171 = local write "Cycle Start Bit"(FALSE ("Cycle Start Bit")) -> ()
        n172 = case shown="True" w262 {
          tunnel: w264 -> [_ w296]
          tunnel: w261 -> [w275 w279]
          tunnel: [w275 w277] -> w260
          frame False {
          }
          frame True {
            n173 = global read "Galobal variable_TI.vi" "Shift Change"() -> (w276:string)
            n174 = stacked-sequence {
              seq-local: [w304 _ _] -> [_ _ w319]
              tunnel: w279 -> [w306 _ _]
              tunnel: [_ _ w319] -> w277
              frame #0 {
                n175 = global read "GR_Servo.vi" "Error Message"() -> (w305:string)
                n176 = case shown="True" TRUE {
                  tunnel: w306 -> [w307 w316]
                  tunnel: w305 -> [_ w311]
                  tunnel: [w307 w308] -> w304
                  frame False {
                  }
                  frame True {
                    n177 = Increment(x=w316) -> (x+1=w308:i32)
                    n178 = Number To Decimal String(number=w308) -> (decimal integer string=w315:string)  [unwired: 1 in]
                    n179 = Bundle By Name(cluster=T15 {"No. Fail Coun t"="", "Rework Status Count 0\\1"="", "NA Count Max =3 "="", "Testesd Count  0/1"="", "Error code"=""} ("Count For Rework"), "No. Fail Coun t"=w315, "Rework Status Count 0\\1"="1" ("Rework Status Count 0\\1"), "NA Count Max =3"="4", "Testesd Count  0/1"="0", "Error code"=w311) -> (w310:T15)
                    n180 = call "Rework Count.vi"("Read /Write"=enum16{"Write", "Read"}."Write", "Count For Rework"=w310) -> ()  [unwired: 8 in, 2 out]
                  }
                }
              }
              frame #1 {
                n181 = Wait (ms)(milliseconds to wait=u32 200) -> ()  [unwired: 1 out]
              }
              frame #2 {
                n182 = global write "Galobal variable_TI.vi" "Rpt Write"(TRUE ("Rpt Write")) -> ()
              }
            }
            n183 = call "Sub_ shift data reset.vi"("Serial no"="NG Counter.txt" ("File Name"), "Shift"=w276, "Model"=w296) -> ("Serial no"=w301:string)  [unwired: 6 in, 1 out]
            n184 = property on="NG Counter" class="Str"("Value"=w301, "Text.BGColor"=u32 16711680 ("Color Box")) -> ()  [unwired: 2 in, 2 out]
            n185 = call <vilib>:"Application Directory.vi"() -> ("Application Directory"=w298:path)
            n186 = Build Path(base path=w298, name or relative path="data\\Report NG") -> (appended path=w299:path)
            n187 = call "Header Create.vi"("File Name"=w296, "path File"=w299) -> ("dup path"=w281:path)  [unwired: 8 in, 1 out]
            n188 = local read "Screw Data(N)"() -> (w291:T2)
            n189 = global read "Galobal variable_TI.vi" "Read LVDT Value"() -> (w289:dbl[])
            n190 = local read "Pokayoka"() -> (w280:T7)
            n191 = local read "Result Lvdt"() -> (w278:T4)
            n192 = Number To Fractional String(number=w289, precision (6)=i16 2) -> (F-format string=w287:string[])  [unwired: 2 in]
            n193 = local read "Running Model"() -> (w293:string)
            n194 = local read "MIC Barcode"() -> (w292:string)
            n195 = local read "User Name"() -> (w294:string)
            n196 = local read "Date time"() -> (w295:string)
            n197 = call "Clip &Lvdt Data.vi"("Pokayoka"=w280, "Result Lvdt in"=w278) -> ("Clip Status"=w286:string, "Screw Height Status"=w285:string)  [unwired: 7 in]
            n198 = Cluster To Array(cluster=w291) -> (array=w290:string[])
            n199 = Build Array (concatenate)(w295, w294, w293, w292, w290, w287, w286, w285) -> (w282:string[])
            n200 = call-poly <vilib>:"Write Delimited Spreadsheet.vi"("file path (dialog if empty)"=w281, "1D data"=w282, "append to file? (F)"=TRUE, "delimiter (\\t)"="," ("delimiter (\\t)")) -> ()  [unwired: 10 in, 2 out]
          }
        }
        n201 = Select(t=AutoTest_seq."Cylender Home" ("Enqueue"), s=w262, f=AutoTest_seq."Error" ("Enqueue")) -> (s? t:f=w265:T1)
        n202 = call "Auotmode.vi"("Enum Selection"=Auot_Test_selection."Enqueue ", "Error In"=w271, "Enqueue"=w265, "queue in"=w273) -> ("error out"=w270:errorcluster, "queue Out"=w272:refnum<queue>)  [unwired: 4 in, 1 out]
      }
      frame "Exit" {
        n203 = global read "Galobal variable_TI.vi" "Manual DO"() -> (w328:bool[])
        n204 = global read "Galobal variable_TI.vi" "Digital input"() -> (w337:bool[])
        n205 = Index Array(array=w337, index #1=14 ("index"), index #2=1 ("index")) -> (element #1=w325:bool, element #2=w324:bool)
        n206 = Replace Array Subset(array=w328, new element #1=FALSE ("new element/subarray"), index #1=4 ("index"), new element #2=TRUE ("new element/subarray"), index #2=5 ("index"), new element #3=FALSE ("new element/subarray"), index #3=10 ("index")) -> (w327:bool[])
        n207 = local write "Start 2"(T6 FALSE ("Start")) -> ()
        n208 = And(x=w325, y=w324) -> (x .and. y?=w323:bool)
        n209 = flat-sequence {
          tunnel: w327 -> [_]
          frame #0 {
            n210 = Wait (ms)(milliseconds to wait=u32 100) -> ()  [unwired: 1 out]
          }
        }
        n211 = global write "Galobal variable_TI.vi" "Manual DO"(w327) -> ()
        n212 = Select(t=AutoTest_seq."Poll Event" ("Enqueue"), s=w323, f=AutoTest_seq."Exit" ("Enqueue")) -> (s? t:f=w332:T1)
        n213 = case shown="True" w325 {
          tunnel: w327 -> [_ _]
          tunnel: [w347 w348] -> w331
          tunnel: w332 -> [w347 w348]
          frame False {
          }
          frame True {
            n214 = call "Tower light.vi"("Enum"=enum16{"Green", "Red", "Yellow"}."Green") -> ()  [unwired: 11 in]
          }
        }
        n215 = global write "GR_Servo.vi" "Error Message"("Home  Button Pressed" ("Error Message")) -> ()
        n216 = call "Auotmode.vi"("Enum Selection"=Auot_Test_selection."Enqueue ", "Enqueue"=w331, "queue in"=w343) -> ("queue Out"=w344:refnum<queue>)  [unwired: 5 in, 2 out]
      }
    }
    n217 = global read "Galobal variable_TI.vi" "Auto Exit"() -> (w84:bool)
  }
  n218 = local write "Start 2"(T6 FALSE ("Start")) -> ()
  n219 = while {
    shift-right: [w389] -> _
    shift-left: w51 -> [w388]
    tunnel: FALSE ("Servo Stop") -> [_]
    tunnel: T8 {"Screw -FL"="", "Screw -FR"="", "Screw -RL"="", "Screw -RR"=""} ("Screw Data(N)") -> [w375]
    stop <- w387 stop-if-true
    # "v"
    n220 = global read "Galobal variable_TI.vi" "Led Enable FL v"() -> (w353:bool)
    n221 = global read "Galobal variable_TI.vi" "Led Enable FR v"() -> (w352:bool)
    n222 = global read "Galobal variable_TI.vi" "Led Enable RR v"() -> (w354:bool)
    n223 = global read "Galobal variable_TI.vi" "Led Enable RL v"() -> (w351:bool)
    n224 = global read "Galobal variable_TI.vi" "NI Comm.Error"() -> (→"Error":bool)
    n225 = global read "Galobal variable_TI.vi" "Result Lvdt"() -> (w366:T13)
    "Result Lvdt" <- w366
    n226 = global read "Galobal variable_TI.vi" "Desontter data 4"() -> (w372:string)
    n227 = global read "Galobal variable_TI.vi" "Desontter data 3"() -> (w370:string)
    n228 = global read "Galobal variable_TI.vi" "Desontter data 2"() -> (w369:string)
    n229 = global read "Galobal variable_TI.vi" "Desontter data1"() -> (w371:string)
    n230 = property on="FL" class="Bool (strict)"("Visible"=w353) -> ()  [unwired: 2 in, 2 out]
    n231 = property on="RR" class="Bool (strict)"("Visible"=w354) -> ()  [unwired: 2 in, 2 out]
    n232 = property on="RL" class="Bool (strict)"("Visible"=w351) -> ()  [unwired: 2 in, 2 out]
    n233 = global write "Galobal variable_TI.vi" "RPT Bypass"("RPT Bypass") -> ()
    n234 = global read "Galobal variable_TI.vi" "LVDT Result bit"() -> (w360:bool)
    n235 = global read "GR_Servo.vi" "ErrorMessage2"() -> (→"Error Message 2":string)
    n236 = property on="FR" class="Bool (strict)"("Visible"=w352) -> ()  [unwired: 2 in, 2 out]
    n237 = Get Date/Time In Seconds() -> (seconds since 1Jan1904=w386:timestamp)
    "Current Date & Time" <- w386
    n238 = Cluster To Array(cluster=w366) -> (array=w365:bool[])
    n239 = Bundle By Name(cluster=w375, "Screw -FL"=w372, "Screw -FR"=w371, "Screw -RL"=w370, "Screw -RR"=w369) -> (→"Screw Data(N)":T8)
    n240 = global read "Galobal variable_TI.vi" "Server"() -> (→"Boolean 2":bool)
    n241 = Select(t=enum32{"Test", "Report"}."Report" ("Tab Control"), s="Report", f=enum32{"Test", "Report"}."Test" ("Tab Control")) -> (s? t:f=w377:enum32{"Test", "Report"})
    n242 = case shown="True" w360 {
      tunnel: w365 -> [_ w401]
      tunnel: [w390 w399] -> w364
      tunnel: [w390 w393] -> w363
      tunnel: [w390 w392] -> w362
      tunnel: [w390 w391] -> w361
      frame False {
        w390 = u32 16448250
      }
      frame True {
        w394 = u32 16711680
        w395 = u32 6618880
        n243 = Index Array(array=w401) -> (element #1=w400:bool, element #2=w398:bool, element #3=w397:bool, element #4=w396:bool)  [unwired: 4 in]
        n244 = Select(t=w395, s=w400, f=w394) -> (s? t:f=w399:u32)
        n245 = Select(t=w395, s=w398, f=w394) -> (s? t:f=w393:u32)
        n246 = Select(t=w395, s=w397, f=w394) -> (s? t:f=w392:u32)
        n247 = Select(t=w395, s=w396, f=w394) -> (s? t:f=w391:u32)
      }
    }
    n248 = local write "Tab Control"(w377) -> ()
    n249 = case shown="False" "Cycle Start Bit" {
      tunnel: w388 -> [_ w404]
      tunnel: w386 -> [w402 w405]
      tunnel: [w402 w404] -> w389
      frame False {
      }
      frame True {
        n250 = Subtract(x=w405, y=w404) -> (x-y=w406:dbl)
        n251 = To Long Integer(number=w406) -> (32bit integer=w403:i32)
        "Cycle Time(Sec)" <- w403
        n252 = local write "Cycle"(w403) -> ()
      }
    }
    n253 = Get Date/Time In Seconds() -> (seconds since 1Jan1904=w383:timestamp)
    n254 = global read "Galobal variable_TI.vi" "Dist. data"() -> (→"Dist. data":dbl[])
    n255 = global read "Galobal variable_TI.vi" "Auto Exit"() -> (w387:bool)
    n256 = Format Date/Time String(time format string (%c)="%d-%m-%Y  %H:%M:%S", seconds (now)=w383) -> (date/time string=→"Date time":string)  [unwired: 1 in]
    n257 = global read "Galobal variable_TI.vi" "Color4"() -> (w358:u32)
    n258 = global read "Galobal variable_TI.vi" "Color1"() -> (w357:u32)
    n259 = global read "Galobal variable_TI.vi" "Color2"() -> (w355:u32)
    n260 = property on="RL" class="Bool (strict)"("BoolText.BGColor"=w355) -> ()  [unwired: 2 in, 2 out]
    n261 = global read "Galobal variable_TI.vi" "Color3"() -> (w356:u32)
    n262 = property on="Screw3(mm)" class="DigNum (strict)"("NumText.BGColor"=w362) -> ()  [unwired: 2 in, 2 out]
    n263 = property on="Screw1(mm)" class="DigNum (strict)"("NumText.BGColor"=w364) -> ()  [unwired: 2 in, 2 out]
    n264 = property on="Screw4(mm)" class="DigNum (strict)"("NumText.BGColor"=w361) -> ()  [unwired: 2 in, 2 out]
    n265 = property on="Screw 2(mm)" class="DigNum (strict)"("NumText.BGColor"=w363) -> ()  [unwired: 2 in, 2 out]
    n266 = global read "Galobal variable_TI.vi" "Running Model"() -> (→"Running Model":string)
    n267 = global read "Galobal variable_TI.vi" "MIC Barcode"() -> (→"MIC Barcode":string)
    n268 = property on="FL" class="Bool (strict)"("BoolText.BGColor"=w357) -> ()  [unwired: 2 in, 2 out]
    n269 = property on="FR" class="Bool (strict)"("BoolText.BGColor"=w356) -> ()  [unwired: 2 in, 2 out]
    n270 = property on="Tightening Torque (Nm)-Screw -RR" class="Str"("Text.BGColor"=w358) -> ()  [unwired: 2 in, 2 out]
    n271 = property on="Tightening Torque(Nm)-Screw -FR" class="Str"("Text.BGColor"=w356) -> ()  [unwired: 2 in, 2 out]
    n272 = property on="Tightening Torque (Nm)-Screw FL" class="Str"("Text.BGColor"=w357) -> ()  [unwired: 2 in, 2 out]
    n273 = property on="Tightening Torque(Nm)- Screw -RL" class="Str"("Text.BGColor"=w355) -> ()  [unwired: 2 in, 2 out]
    n274 = property on="RR" class="Bool (strict)"("BoolText.BGColor"=w358) -> ()  [unwired: 2 in, 2 out]
  }
  n275 = call "Desonatter Torque data read.vi"() -> ()  [unwired: 9 in, 3 out]
  n276 = call "screw empty message.vi"() -> ()  [unwired: 12 in]
  n277 = while {
    stop <- w408 stop-if-true
    n278 = event shown="[0] Timeout" {
      selector: _ -> [_ _]
      dyn-events: _ -> [_ _]
      timeout: 2 -> [_ _]
      event Timeout {
        n279 = event-data() -> ()  [unwired: 1 in, 3 out]
        n280 = global read "Galobal variable_TI.vi" "Digital input"() -> (w415:bool[])
        n281 = call "Sensor Poka Yoka.vi"("Digital input"=w415) -> ("Pokayoka"=w436:T7)  [unwired: 9 in]
        "Pokayoka" <- w436
        n282 = Unbundle By Name(w436) -> ("Clip1"=w435:bool, "Clip2 3"=w433:bool, "Clip3 3"=w432:bool, "Clip4"=w429:bool, "Clip5"=w427:bool, "Clip6"=w425:bool, "Clip7"=w423:bool, "Clip8"=w421:bool)
        n283 = Not(x=w435) -> (.not. x?=w434:bool)
        n284 = Not(x=w427) -> (.not. x?=w426:bool)
        n285 = Not(x=w433) -> (.not. x?=w431:bool)
        n286 = Not(x=w432) -> (.not. x?=w430:bool)
        n287 = Not(x=w425) -> (.not. x?=w424:bool)
        n288 = Not(x=w429) -> (.not. x?=w428:bool)
        n289 = property on="Clip1" class="Bool (strict)"("Blinking"=w434) -> ()  [unwired: 2 in, 2 out]
        n290 = property on="Clip2 3" class="Bool (strict)"("Blinking"=w431) -> ()  [unwired: 2 in, 2 out]
        n291 = property on="Clip3 3" class="Bool (strict)"("Blinking"=w430) -> ()  [unwired: 2 in, 2 out]
        n292 = property on="Clip4" class="Bool (strict)"("Blinking"=w428) -> ()  [unwired: 2 in, 2 out]
        n293 = property on="Clip5" class="Bool (strict)"("Blinking"=w426) -> ()  [unwired: 2 in, 2 out]
        n294 = property on="Clip6" class="Bool (strict)"("Blinking"=w424) -> ()  [unwired: 2 in, 2 out]
        n295 = Not(x=w423) -> (.not. x?=w422:bool)
        n296 = Index Array(array=w415, index #1=8 ("index"), index #2=9 ("index")) -> (element #1=w441:bool, element #2=w444:bool)
        n297 = Index Array(array=w415, index=16) -> (element=w413:bool)
        n298 = Index Array(array=w415, index #2=31 ("index")) -> (element #1=→"Servo Fault":bool, element #2=w448:bool)  [unwired: 1 in]
        n299 = property on="Clip7" class="Bool (strict)"("Blinking"=w422) -> ()  [unwired: 2 in, 2 out]
        n300 = Not(x=w421) -> (.not. x?=w420:bool)
        n301 = Or(x=w441, y=w444) -> ()  [unwired: 1 out]
        n302 = case shown="False" w441 {
          tunnel: w444 -> [w463 _]
          tunnel: w441 -> [_ w466]
          frame False {
            n303 = case shown="True" w463 {
              tunnel: w463 -> [_ w464]
              frame False {
              }
              frame True {
                n304 = global write "Galobal variable_TI.vi" "DC OK"(FALSE ("DC OK")) -> ()
                n305 = global write "Galobal variable_TI.vi" "DCNG"(w464) -> ()
              }
            }
          }
          frame True {
            n306 = global write "Galobal variable_TI.vi" "DC OK"(w466) -> ()
            n307 = global write "Galobal variable_TI.vi" "DCNG"(FALSE ("DCNG")) -> ()
          }
        }
        n308 = Index Array(array=w415, index #1=0 ("index"), index #2=8 ("index"), index #3=2 ("index"), index #4=18 ("index")) -> (element #1=→"Start":bool, element #2=w457:bool, element #3=→"reset":bool, element #4=→"Proxi Sensor":bool)
        n309 = global read "Galobal variable_TI.vi" "Ring Sensor Off  Bit"() -> (w447:bool)
        n310 = property on="Clip8" class="Bool (strict)"("Blinking"=w420) -> ()  [unwired: 2 in, 2 out]
        n311 = case shown="True" w413 {
          frame False {
          }
          frame True {
          }
        }
        n312 = global read "Galobal variable_TI.vi" "STM Done Bit"() -> (w458:bool)
        n313 = global read "Galobal variable_TI.vi" "Manual DO"() -> (w416:bool[])
        n314 = global read "Galobal variable_TI.vi" "Read LVDT Value"() -> (w443:dbl[])
        "Read LVDT Value" <- w443
        n315 = Replace Array Subset(array=w416, new element=TRUE ("Feeder"), index=25) -> (w419:bool[])
        n316 = case shown="False" w448 {
          tunnel: w448 -> [_ w470]
          tunnel: w447 -> [w468 _]
          frame False {
            n317 = case shown="True" w468 {
              frame False {
              }
              frame True {
                n318 = global write "Galobal variable_TI.vi" "Ring Sensor On Bit"(FALSE ("Ring Sensor")) -> ()
              }
            }
          }
          frame True {
            n319 = global write "Galobal variable_TI.vi" "Ring Sensor On Bit"(w470) -> ()
          }
        }
        n320 = global read "Galobal variable_TI.vi" "Feeder Empty"() -> (w412:bool)
        n321 = global write "Galobal variable_TI.vi" "Manual DO"(w419) -> ()
        n322 = global read "GR_Servo.vi" "Error Message"() -> (w411:string)
        n323 = Array To Cluster(array=w443) -> (cluster=→"Result Lvdt 2":T17)
        n324 = Select(t="Screw Feeder Empty/Screw Stuck In Feeder", s=w412, f=w411) -> (s? t:f=→"Error Message":string)
        n325 = global read "Galobal variable_TI.vi" "Led Enable FL"() -> (→"FL":bool)
        n326 = global read "Galobal variable_TI.vi" "Led Enable RR"() -> (→"RR":bool)
        n327 = global read "Galobal variable_TI.vi" "Led Enable RL"() -> (→"RL":bool)
        n328 = global read "Galobal variable_TI.vi" "Led Enable FR"() -> (→"FR":bool)
        n329 = Or(x=w457, y=w458) -> (x .or. y?=w456:bool)
        n330 = Select(t=cluster{u32, u32}[] [{16734762, 6618880}, {16777222, 6618880}] ("Colors [4]"), s=w456, f=cluster{u32, u32}[] [{16734762, 16711680}, {16777222, 16775560}] ("Colors [4]")) -> ()  [unwired: 1 out]
      }
      event Value Change {
        n331 = event-data() -> ("NewVal"=w471:T5)  [unwired: 1 in]
        n332 = global write "Galobal variable_TI.vi" "Auto Exit"(w471) -> ()
        n333 = global read "Galobal variable_TI.vi" "Digital input"() -> (→"DI":bool[])
      }
    }
    n334 = local read "Exit"() -> (w408:T5)
  }
  n335 = disable-structure shown="Disabled" {
    frame Disabled {
      w473 = FALSE
      n336 = global write "Galobal variable_TI.vi" "Led Enable RR"(w473) -> ()
      n337 = global write "Galobal variable_TI.vi" "Led Enable RR"(w473) -> ()
      n338 = global write "Galobal variable_TI.vi" "Led Enable RR"(w473) -> ()
      n339 = global write "Galobal variable_TI.vi" "Led Enable RR"(w473) -> ()
    }
    frame Enabled {
    }
  }
  n340 = disable-structure shown="Disabled" {
    frame Disabled {
      n341 = global read "Galobal variable_TI.vi" "Manual DO"() -> ()  [unwired: 1 out]
    }
    frame Enabled {
    }
  }
  n342 = disable-structure shown="Disabled" {
    frame Disabled {
    }
    frame Enabled {
    }
  }
  n343 = call "Auotmode.vi"("Enum Selection"=Auot_Test_selection."Flush", "Error In"=w45, "queue in"=w52) -> ("error out"=w57:errorcluster, "queue Out"=w56:refnum<queue>)  [unwired: 5 in, 1 out]
  n344 = call "Auotmode.vi"("Enum Selection"=Auot_Test_selection."Release Queue", "Error In"=w57, "queue in"=w56) -> ("error out"=→"error out":errorcluster)  [unwired: 5 in, 2 out]
